vi "Test Configurable Buffer.vi"() -> ()   [LabVIEW 2016]
uses:
  Configurable Buffer.xctl
panel:
  out "MFC":cluster{"Val":dbl[], "time":timestamp}(xcontrol) caption="Configurable Buffer"
  out "Velocity":cluster{"Val":dbl[], "time":timestamp}(xcontrol) caption="Configurable Buffer"
  out "Vaisala":cluster{"Val":dbl[], "time":timestamp}(xcontrol) caption="Configurable Buffer"
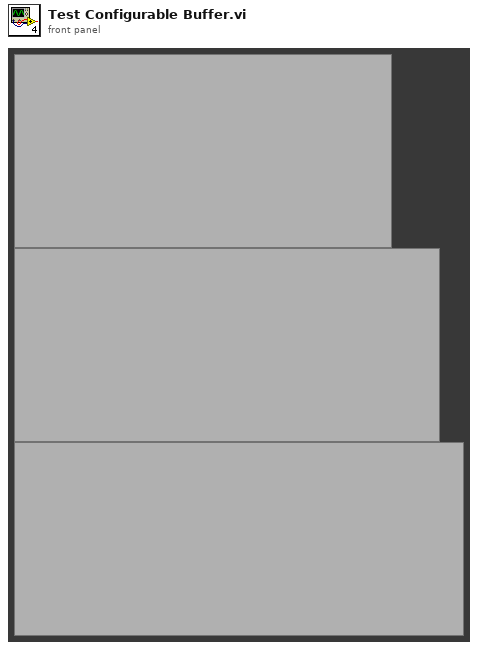
[diagram p1: front panel]
types:
  T1 = cluster{dbl[], "seconds since 1Jan1904":timestamp}
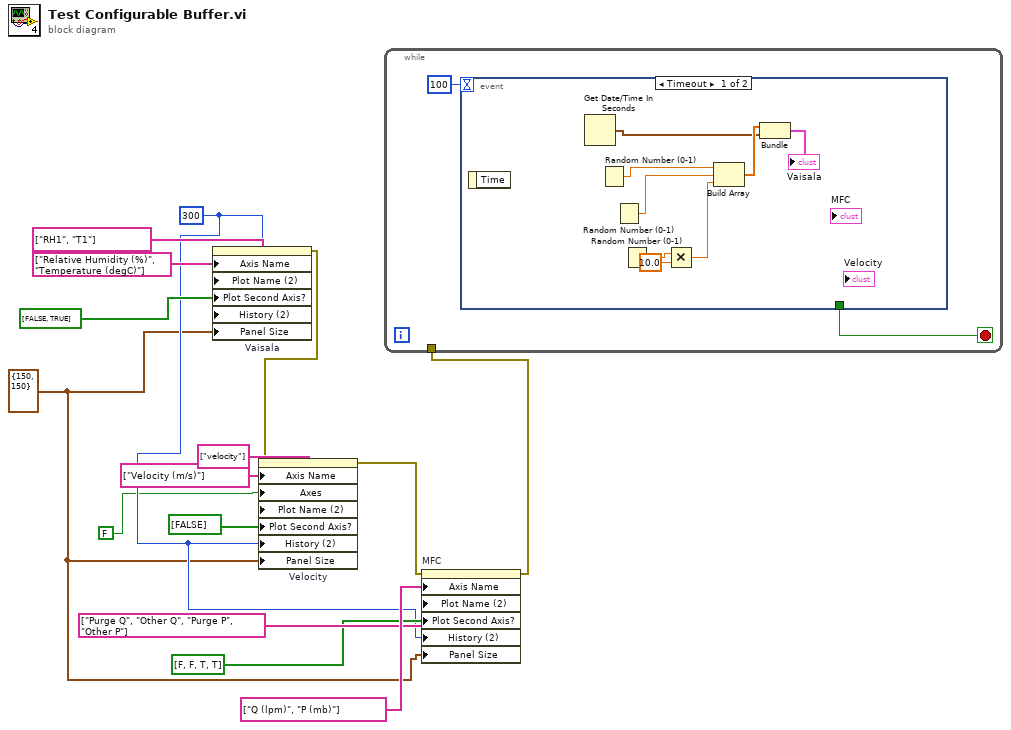
[diagram p0: block diagram]
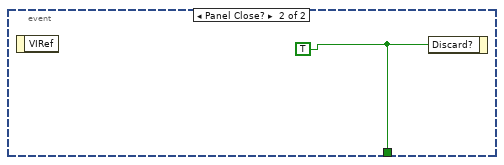
[diagram p2: hidden frame]
diagram:
  w5 = cluster{"Height":i16, "Width":i16} {"Height"=150, "Width"=150} ("Panel Size")
  w6 = 300 ("History")
  n1 = property on="Vaisala" class="Configurable Buffer (strict)"("Axis Name"=string[] ["Relative Humidity (%)", "Temperature (degC)"], "Plot Name (2)"=string[] ["RH1", "T1"] ("Plot Name"), "Plot Second Axis?"=bool[] [FALSE, TRUE], "History (2)"=w6, "Panel Size"=w5) -> (error out=w4:errorcluster)  [unwired: 2 in, 1 out]
  n2 = property on="Velocity" class="Configurable Buffer (strict)"(error in=w4, "Axis Name"=string[] ["Velocity (m/s)"], "Axes"=FALSE ("Two Axes?"), "Plot Name (2)"=string[] ["velocity"] ("Plot Name"), "Plot Second Axis?"=bool[] [FALSE], "History (2)"=w6, "Panel Size"=w5) -> (error out=w3:errorcluster)  [unwired: 1 in, 1 out]
  n3 = property on="MFC" class="Configurable Buffer (strict)"(error in=w3, "Axis Name"=string[] ["Q (lpm)", "P (mb)"], "Plot Name (2)"=string[] ["Purge Q", "Other Q", "Purge P", "Other P"] ("Plot Name"), "Plot Second Axis?"=bool[] [FALSE, FALSE, TRUE, TRUE], "History (2)"=w6, "Panel Size"=w5) -> (error out=w2:errorcluster)  [unwired: 1 in, 1 out]
  n4 = while {
    tunnel: w2 -> [_]
    stop <- w17 stop-if-true
    n5 = event shown="[0] Timeout" {
      selector: _ -> [_ _]
      dyn-events: _ -> [_ _]
      timeout: 100 -> [_ _]
      tunnel: [_ w26] -> w17
      event Timeout {
        n6 = event-data() -> ()  [unwired: 1 in, 1 out]
        n7 = Get Date/Time In Seconds() -> (seconds since 1Jan1904=w19:timestamp)
        n8 = Random Number (0-1)() -> (number: 0 to 1=w23:dbl)
        n9 = Random Number (0-1)() -> (number: 0 to 1=w22:dbl)
        n10 = Random Number (0-1)() -> (number: 0 to 1=w25:dbl)
        n11 = Multiply(x=w25, y=10.0) -> (x*y=w21:dbl)
        n12 = Build Array(w23, w22, w21) -> (w20:dbl[])
        n13 = Bundle(w20, "seconds since 1Jan1904"=w19) -> (→"Vaisala":T1)  [unwired: 1 in]
      }
      event Panel Close? {
        w26 = TRUE
        n14 = event-data() -> ()  [unwired: 1 in, 1 out]
        n15 = event-data("Discard?"=w26) -> ()  [unwired: 1 in, 1 out]
      }
    }
  }
